vi "Deserialise content.vi"(8 "error in (no error)":errorcluster, 10 "JSON String to decode":string, 11 "object in":refnum<class "Reply Message.lvclass">) -> (0 "error out":errorcluster, 3 "object out":refnum<class "Reply Message.lvclass">)   [LabVIEW 2018, in "ClientMessaging.lvlib" / "Reply Message.lvclass"]
uses:
  Reply Message.lvclass
  Message Class/Message Class.lvclass
  21d936e0-9587-4355-97ac-c4ab148bb4c4.vi
  160358ff-c91a-4a5a-aaf0-729cc1991d9b.vi
  bc4ebbc4-67bf-4239-a22e-b8cdcd86b670.vi
  f9218fa9-97f6-43c8-a721-e8dd93e9015f.vi
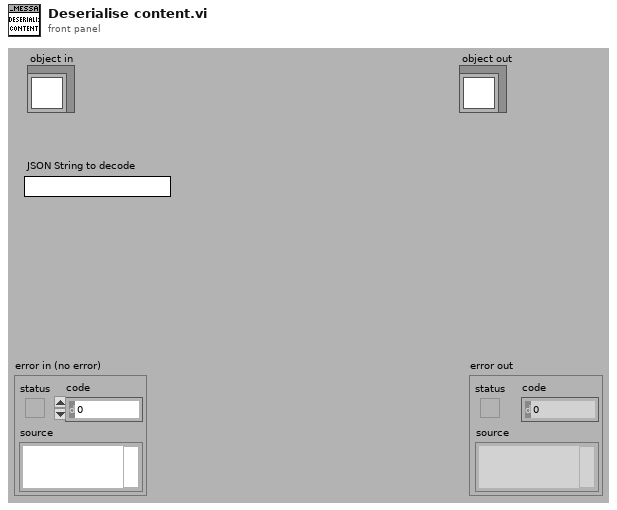
[diagram p1: front panel]
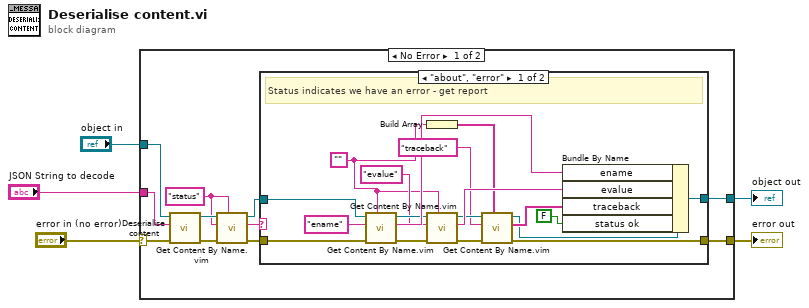
[diagram p0: block diagram]
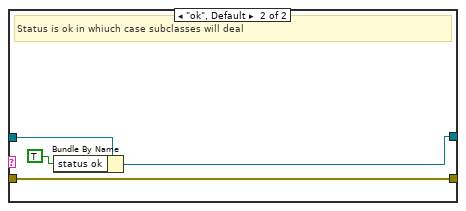
[diagram p2: hidden frame]
diagram:
  n1 = case shown="No Error" "error in (no error)" {
    selector: "error in (no error)" -> [w12 w40]
    tunnel: [w15 w40] -> w4
    tunnel: [w16 w39] -> w2
    tunnel: "object in" -> [w14 w39]
    tunnel: "JSON String to decode" -> [w13 _]
    frame No Error {
      w6 = "status"
      n2 = call-parent "Deserialise content.vi"("error in (no error)"=w12, "JSON String to decode"=w13, "object in"=w14) -> ("error out"=w10:errorcluster, "object out"=w11:refnum<class "Reply Message.lvclass">)  [unwired: 7 in]
      n3 = call "Get Content By Name.vim"("Type of content"=w6, "error in (no error)"=w10, "Name of Content Item"=w6, "Message In"=w11) -> ("error out"=w7:errorcluster, "Data Out"=w9:string, "Message Out"=w8:refnum<class "Reply Message.lvclass">)  [unwired: 5 in]
      n4 = case shown="\"about\", \"error\"" w9 {
        tunnel: [w34 w36] -> w16
        tunnel: [w20 w38] -> w15
        tunnel: w7 -> [w18 w38]
        tunnel: w8 -> [w33 w37]
        frame "about", "error" {
          w27 = ""
          # "Status indicates we have an error - get report"
          n5 = call "Get Content By Name.vim"("Type of content"=w27, "error in (no error)"=w18, "Name of Content Item"="ename" ("Element Name"), "Message In"=w33) -> ("error out"=w29:errorcluster, "Data Out"=w31:string, "Message Out"=w30:refnum<class "Reply Message.lvclass">)  [unwired: 5 in]
          n6 = Build Array(w27) -> (w22:string[])
          n7 = call "Get Content By Name.vim"("Type of content"=w27, "error in (no error)"=w29, "Name of Content Item"="evalue" ("Element Name"), "Message In"=w30) -> ("error out"=w24:errorcluster, "Data Out"=w26:string, "Message Out"=w25:refnum<class "Reply Message.lvclass">)  [unwired: 5 in]
          n8 = call "Get Content By Name.vim"("Type of content"=w22, "error in (no error)"=w24, "Name of Content Item"="traceback" ("Element Name"), "Message In"=w25) -> ("error out"=w20:errorcluster, "Data Out"=w21:string[], "Message Out"=w19:refnum<class "Reply Message.lvclass">)  [unwired: 5 in]
          n9 = Bundle By Name(cluster=w19, "ename"=w31, "evalue"=w26, "traceback"=w21, "status ok"=FALSE) -> (w34:refnum<class "Reply Message.lvclass">)
        }
        frame "ok", Default {
          # "Status is ok in whiuch case subclasses will deal"
          n10 = Bundle By Name(cluster=w37, "status ok"=TRUE) -> (w36:refnum<class "Reply Message.lvclass">)
        }
      }
    }
    frame Error {
    }
  }
  "error out" <- w4
  "object out" <- w2
